vi "Pulse.vi"(8 "error in (no error)":errorcluster, 9 "Sender":string, 10 "Pulse In":enum16{"Low", "High"}(ring), 11 "Flip Flop In":refnum<class "Flip Flop.lvclass">) -> (0 "error out":errorcluster, 1 "Receivers":string[](array[string]), 2 "Pulse Out":enum16{"Low", "High"}(ring), 3 "Flip Flop Out":refnum<class "Flip Flop.lvclass">)   [LabVIEW 2021, in "Flip Flop.lvclass"]
uses:
  Flip Flop.lvclass
  Flip Flop.lvclass/Flip Flop.ctl
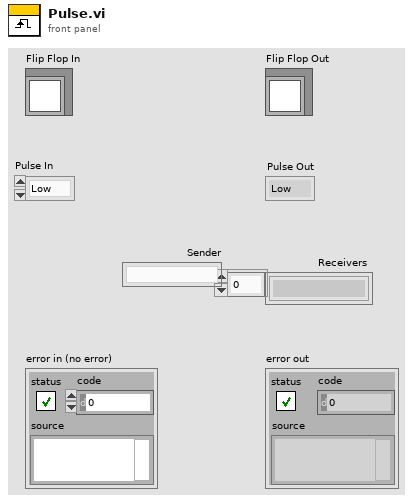
[diagram p1: front panel]
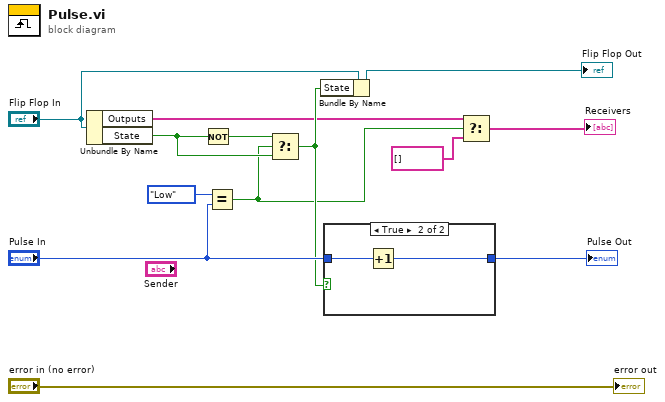
[diagram p0: block diagram]
diagram:
  n1 = Unbundle By Name("Flip Flop In") -> ("Outputs"=w2:string[], "State"=w6:bool)
  n2 = Not(x=w6) -> (.not. x?=w7:bool)
  n3 = Equal?(x=enum16{"Low", "High"}."Low", y="Pulse In") -> (x = y?=w4:bool)
  n4 = Select(t=w7, s=w4, f=w6) -> (s? t:f=w5:bool)
  n5 = Bundle By Name(cluster="Flip Flop In", "State"=w5) -> (→"Flip Flop Out":refnum<class "Flip Flop.lvclass">)
  n6 = case shown="True" w5 {
    tunnel: "Pulse In" -> [w14 w16]
    tunnel: [w14 w15] -> w11
    frame False {
    }
    frame True {
      n7 = Increment(x=w16) -> (x+1=w15:enum16{"Low", "High"})
    }
  }
  "Pulse Out" <- w11
  n8 = Select(t=w2, s=w4, f=string[] []) -> (s? t:f=→"Receivers":string[])
  "error out" <- "error in (no error)"
